vi "FTW-ERR-NoErrorConstant.vi"() -> (0 "no error":errorcluster)   [LabVIEW 2013, in "XML.lvlib"]
uses:
  XML.lvlib
panel:
  # "Outputs"
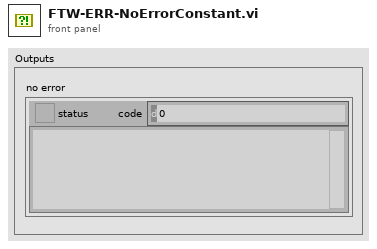
[diagram p1: front panel]
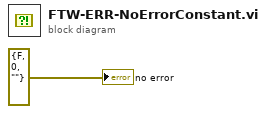
[diagram p0: block diagram]
diagram:
  "no error" <- errorcluster {"status"=FALSE, "code"=0, "source"=""} ("no error")
